vi "Configure Hardware.vi"(8 "error in (no error)":errorcluster, 11 "Hardware Resources in":T1={"AI"={"DAQmx Channel"="", "Max Input"=0.0, "Min Input"=0.0, "Sample Rate"=0.0, "DAQmx Task"="", "shunt resistor location"=-1, "external shunt resistor value"=249.0}, "AO"={"DAQmx Channel"="", "Max Output"=0.0, "Min Output"=0.0, "Sample Rate"=0.0, "DAQmx Task"=""}, "DO"={"DAQmx Channel"="", "Sample Rate"=0.0, "DAQmx Task"=""}, "DI"={"DAQmx Channel"="", "Sample Rate"=0.0, "DAQmx Task"=""}, "TC"={"DAQmx Channel"="", "Max Inout"=0.0, "Min Input"=0.0, "Sample Rate"=0.0, "DAQmx Task"="", "resistance configuration"=4, "r0"=100.0, "current excitation value"=0.0025, "current excitation source"=10167, "rtd type"=12481}} {"TC"."rtd type" items=["Pt3750"=12481, "Pt3851"=10071, "Pt3911"=12482, "Pt3916"=10069, "Pt3920"=10053, "Pt3928"=12483, "Custom"=10137]; "TC"."current excitation source" items=["Internal"=10200, "External"=10167, "None"=10230]; "TC"."resistance configuration" items=["2-Wire"=2, "3-Wire"=3, "4-Wire"=4]; "AI"."shunt resistor location" items=["default"=-1, "RSE"=10083, "NRSE"=10078, "Differential"=10106, "Pseudodifferential"=12529]}) -> (0 "error out":errorcluster, 3 "Hardware Resources out":T1={"AI"={"DAQmx Channel"="", "Max Input"=0.0, "Min Input"=0.0, "Sample Rate"=0.0, "DAQmx Task"="", "shunt resistor location"=-1, "external shunt resistor value"=249.0}, "AO"={"DAQmx Channel"="", "Max Output"=0.0, "Min Output"=0.0, "Sample Rate"=0.0, "DAQmx Task"=""}, "DO"={"DAQmx Channel"="", "Sample Rate"=0.0, "DAQmx Task"=""}, "DI"={"DAQmx Channel"="", "Sample Rate"=0.0, "DAQmx Task"=""}, "TC"={"DAQmx Channel"="", "Max Inout"=0.0, "Min Input"=0.0, "Sample Rate"=0.0, "DAQmx Task"="", "resistance configuration"=4, "r0"=100.0, "current excitation value"=0.0025, "current excitation source"=10167, "rtd type"=12481}} {"TC"."rtd type" items=["Pt3750"=12481, "Pt3851"=10071, "Pt3911"=12482, "Pt3916"=10069, "Pt3920"=10053, "Pt3928"=12483, "Custom"=10137]; "TC"."current excitation source" items=["Internal"=10200, "External"=10167, "None"=10230]; "TC"."resistance configuration" items=["2-Wire"=2, "3-Wire"=3, "4-Wire"=4]; "AI"."shunt resistor location" items=["default"=-1, "RSE"=10083, "NRSE"=10078, "Differential"=10106, "Pseudodifferential"=12529]})   [LabVIEW 2024, in "Acquisition.lvlib"]
doc: "Configure the hardware."
uses:
  Acquisition.lvlib
  Hardware Configuration.ctl
  <vilib>/DAQmx/configure/timing.llb/DAQmx Timing (Sample Clock).vi
  <vilib>/DAQmx/create/channels.llb/DAQmx Create Channel (DI-Digital Input).vi
  <vilib>/DAQmx/create/channels.llb/DAQmx Create Channel (AO-Current-Basic).vi
  <vilib>/DAQmx/create/channels.llb/DAQmx Create Channel (DO-Digital Output).vi
  <vilib>/DAQmx/create/channels.llb/DAQmx Create Channel (AI-Temperature-RTD).vi
  <vilib>/DAQmx/create/channels.llb/DAQmx Create Channel (AI-Current-Basic).vi
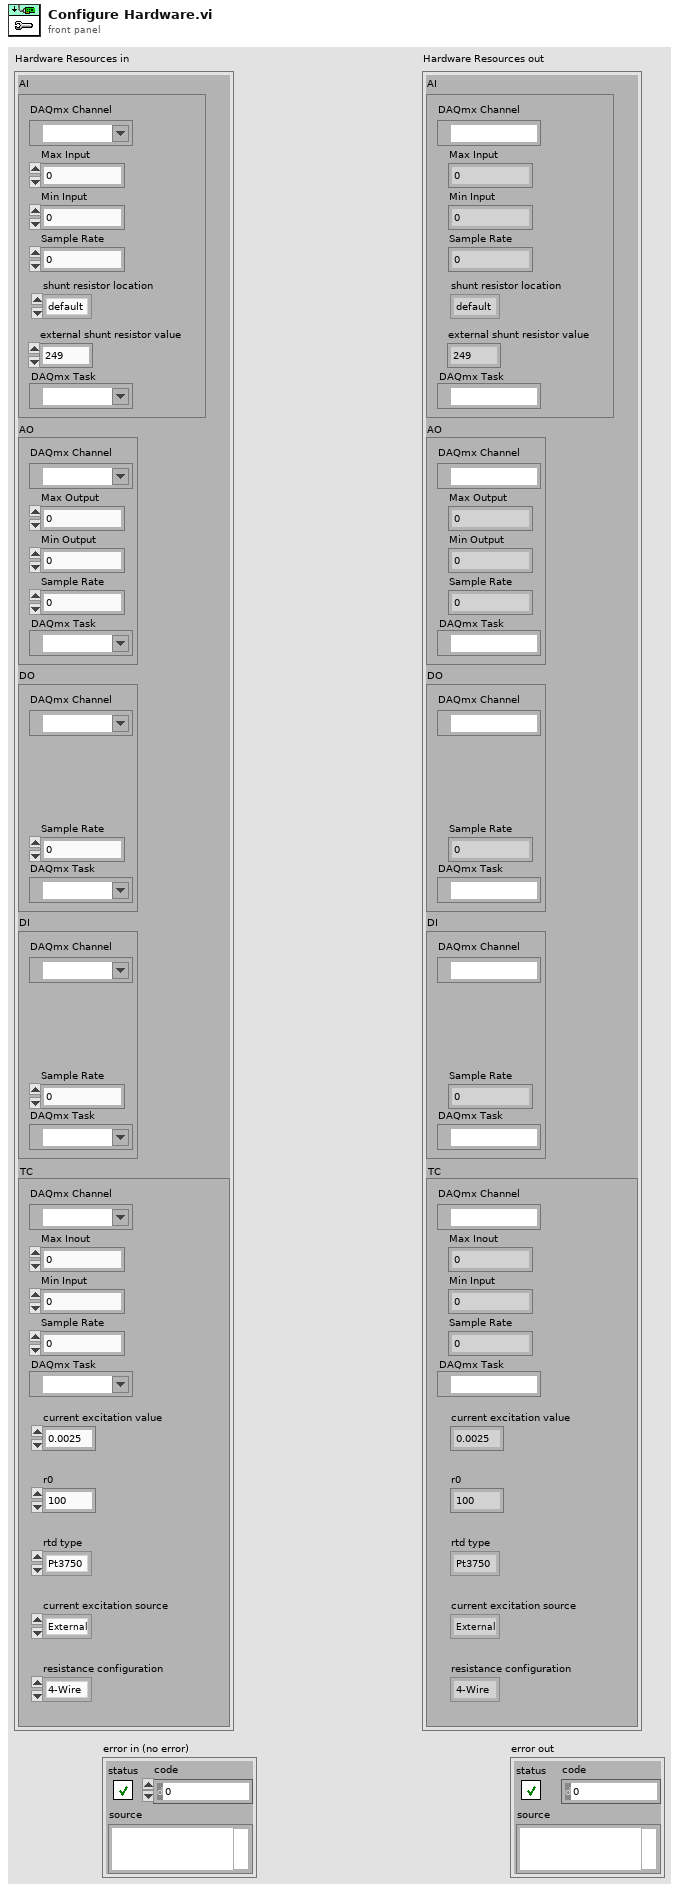
[diagram p1: front panel]
types:
  T1 = typedef "Acquisition.lvlib/Hardware Configuration.ctl" = cluster{"AI":cluster{"DAQmx Channel":tag, "Max Input":dbl, "Min Input":dbl, "Sample Rate":dbl, "DAQmx Task":refnum<k21>, "shunt resistor location":i32, "external shunt resistor value":dbl}, "AO":cluster{"DAQmx Channel":tag, "Max Output":dbl, "Min Output":dbl, "Sample Rate":dbl, "DAQmx Task":refnum<k21>}, "DO":cluster{"DAQmx Channel":tag, "Sample Rate":dbl, "DAQmx Task":refnum<k21>}, "DI":cluster{"DAQmx Channel":tag, "Sample Rate":dbl, "DAQmx Task":refnum<k21>}, "TC":cluster{"DAQmx Channel":tag, "Max Inout":dbl, "Min Input":dbl, "Sample Rate":dbl, "DAQmx Task":refnum<k21>, "resistance configuration":i32, "r0":dbl, "current excitation value":dbl, "current excitation source":i32, "rtd type":i32}}
  T2 = cluster{"DAQmx Channel":tag, "Max Input":dbl, "Min Input":dbl, "Sample Rate":dbl, "DAQmx Task":refnum<k21>, "shunt resistor location":i32, "external shunt resistor value":dbl}
  T3 = cluster{"DAQmx Channel":tag, "Max Output":dbl, "Min Output":dbl, "Sample Rate":dbl, "DAQmx Task":refnum<k21>}
  T4 = cluster{"DAQmx Channel":tag, "Sample Rate":dbl, "DAQmx Task":refnum<k21>}
  T5 = cluster{"DAQmx Channel":tag, "Max Inout":dbl, "Min Input":dbl, "Sample Rate":dbl, "DAQmx Task":refnum<k21>, "resistance configuration":i32, "r0":dbl, "current excitation value":dbl, "current excitation source":i32, "rtd type":i32}
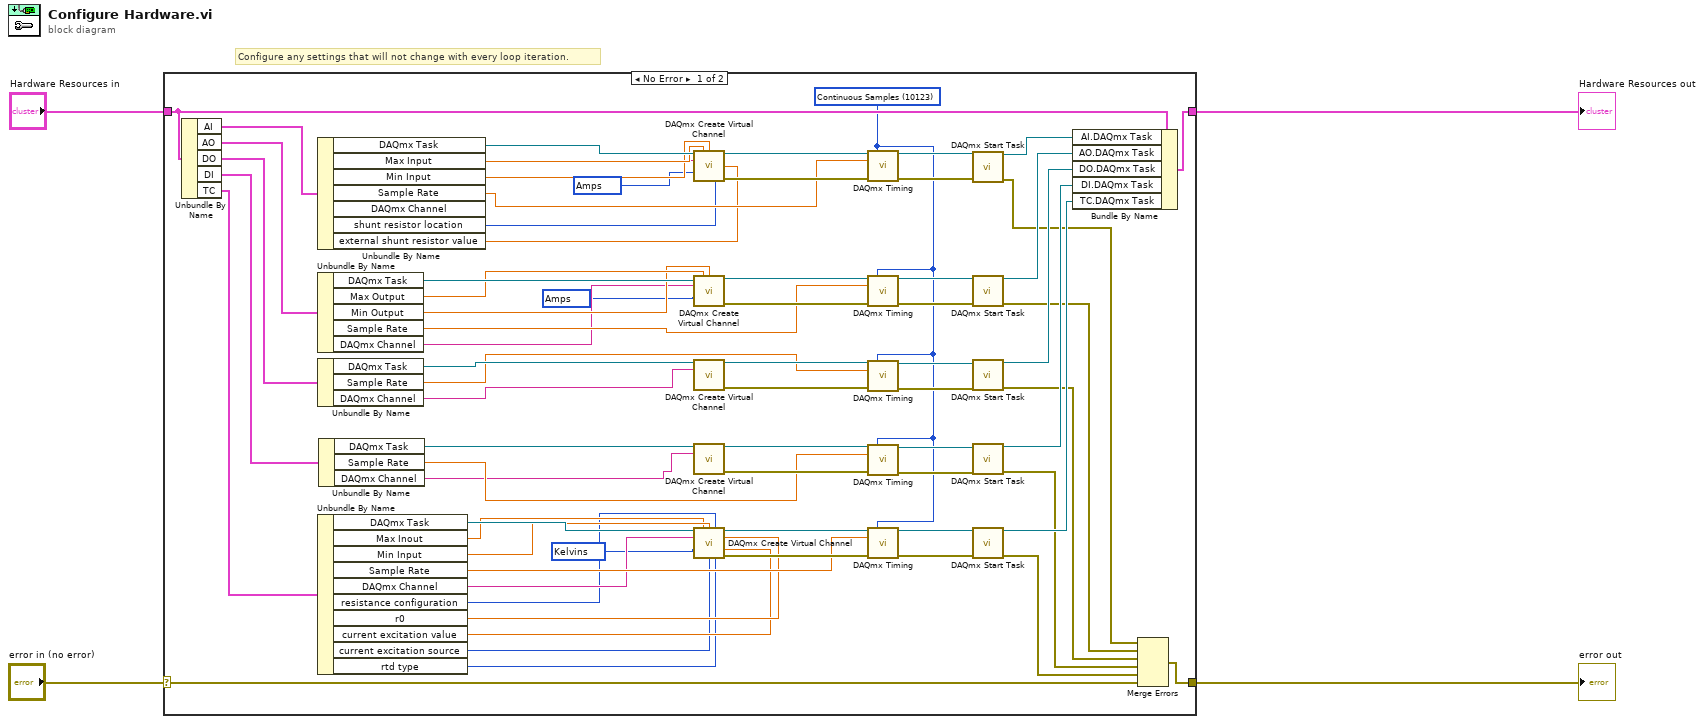
[diagram p0: block diagram]
diagram:
  # "Configure any settings that will not change with every loop iteration."
  n1 = case shown="No Error" "error in (no error)" {
    selector: "error in (no error)" -> [w59 w76]
    tunnel: [w8 w76] -> w3
    tunnel: "Hardware Resources in" -> [w53 w77]
    tunnel: [w75 w77] -> w2
    frame No Error {
      w5 = 10342 items=["Amps"=10342, "From Custom Scale"=10065] ("units")
      w6 = 10342 items=["Amps"=10342, "From Custom Scale"=10065] ("units")
      w7 = 10325 items=["Deg C"=10143, "Deg F"=10144, "Kelvins"=10325, "Deg R"=10145, "From Custom Scale"=10065] ("units")
      w14 = 10123 items=["Finite Samples"=10178, "Continuous Samples"=10123, "Hardware Timed Single Point"=12522] ("sample mode")
      n2 = Unbundle By Name(w53) -> ("AI"=w48:T2, "AO"=w49:T3, "DO"=w50:T4, "DI"=w51:T4, "TC"=w52:T5)
      n3 = Unbundle By Name(w48) -> ("DAQmx Task"=w37:refnum<k21>, "Max Input"=w32:dbl, "Min Input"=w31:dbl, "Sample Rate"=w30:dbl, "DAQmx Channel"=w29:tag, "shunt resistor location"=w28:i32, "external shunt resistor value"=w27:dbl)
      n4 = Unbundle By Name(w49) -> ("DAQmx Task"=w36:refnum<k21>, "Max Output"=w26:dbl, "Min Output"=w25:dbl, "Sample Rate"=w24:dbl, "DAQmx Channel"=w23:tag)
      n5 = Unbundle By Name(w50) -> ("DAQmx Task"=w35:refnum<k21>, "Sample Rate"=w22:dbl, "DAQmx Channel"=w21:tag)
      n6 = Unbundle By Name(w52) -> ("DAQmx Task"=w33:refnum<k21>, "Max Inout"=w17:dbl, "Min Input"=w18:dbl, "Sample Rate"=w16:dbl, "DAQmx Channel"=w15:tag, "resistance configuration"=w13:i32, "r0"=w12:dbl, "current excitation value"=w11:dbl, "current excitation source"=w10:i32, "rtd type"=w9:i32)
      n7 = Unbundle By Name(w51) -> ("DAQmx Task"=w34:refnum<k21>, "Sample Rate"=w20:dbl, "DAQmx Channel"=w19:tag)
      n8 = call-poly <vilib>:"DAQmx Create Virtual Channel.vi"("task in"=w37, "maximum value"=w32, "minimum value"=w31, "physical channels"=w29, "external shunt resistor value"=w27, "units"=w5, "shunt resistor location"=w28) -> ("task out"=w47:refnum<k21>, "error out"=w42:errorcluster)  [unwired: 7 in]
      n9 = call-poly <vilib>:"DAQmx Create Virtual Channel.vi"("task in"=w36, "maximum value"=w26, "minimum value"=w25, "physical channels"=w23, "units"=w6) -> ("task out"=w45:refnum<k21>, "error out"=w41:errorcluster)  [unwired: 9 in]
      n10 = call-poly <vilib>:"DAQmx Create Virtual Channel.vi"("task in"=w35, "lines"=w21) -> ("task out"=w44:refnum<k21>, "error out"=w40:errorcluster)  [unwired: 12 in]
      n11 = call-poly <vilib>:"DAQmx Create Virtual Channel.vi"("task in"=w34, "lines"=w19) -> ("task out"=w43:refnum<k21>, "error out"=w39:errorcluster)  [unwired: 12 in]
      n12 = call-poly <vilib>:"DAQmx Create Virtual Channel.vi"("task in"=w33, "maximum value"=w17, "minimum value"=w18, "resistance configuration"=w13, "physical channels"=w15, "r0"=w12, "units"=w7, "current excitation value"=w11, "current excitation source"=w10, "rtd type"=w9) -> ("task out"=w46:refnum<k21>, "error out"=w38:errorcluster)  [unwired: 4 in]
      n13 = call-poly <vilib>:"DAQmx Timing.vi"("task/channels in"=w47, "sample mode"=w14, "rate"=w30, "error in"=w42) -> ("task out"=w69:refnum<k21>, "error out"=w64:errorcluster)  [unwired: 10 in]
      n14 = call-poly <vilib>:"DAQmx Timing.vi"("task/channels in"=w45, "sample mode"=w14, "rate"=w24, "error in"=w41) -> ("task out"=w65:refnum<k21>, "error out"=w63:errorcluster)  [unwired: 10 in]
      n15 = call-poly <vilib>:"DAQmx Timing.vi"("task/channels in"=w44, "sample mode"=w14, "rate"=w22, "error in"=w40) -> ("task out"=w66:refnum<k21>, "error out"=w62:errorcluster)  [unwired: 10 in]
      n16 = call-poly <vilib>:"DAQmx Timing.vi"("task/channels in"=w43, "sample mode"=w14, "rate"=w20, "error in"=w39) -> ("task out"=w67:refnum<k21>, "error out"=w61:errorcluster)  [unwired: 10 in]
      n17 = call-poly <vilib>:"DAQmx Timing.vi"("task/channels in"=w46, "sample mode"=w14, "rate"=w16, "error in"=w38) -> ("task out"=w68:refnum<k21>, "error out"=w60:errorcluster)  [unwired: 10 in]
      n18 = call <vilib>:"DAQmx Start Task.vi"("task/channels in"=w69, "error in"=w64) -> ("task out"=w74:refnum<k21>, "error out"=w54:errorcluster)  [unwired: 12 in]
      n19 = call <vilib>:"DAQmx Start Task.vi"("task/channels in"=w65, "error in"=w63) -> ("task out"=w73:refnum<k21>, "error out"=w55:errorcluster)  [unwired: 12 in]
      n20 = call <vilib>:"DAQmx Start Task.vi"("task/channels in"=w66, "error in"=w62) -> ("task out"=w72:refnum<k21>, "error out"=w56:errorcluster)  [unwired: 12 in]
      n21 = call <vilib>:"DAQmx Start Task.vi"("task/channels in"=w67, "error in"=w61) -> ("task out"=w71:refnum<k21>, "error out"=w57:errorcluster)  [unwired: 12 in]
      n22 = call <vilib>:"DAQmx Start Task.vi"("task/channels in"=w68, "error in"=w60) -> ("task out"=w70:refnum<k21>, "error out"=w58:errorcluster)  [unwired: 12 in]
      n23 = Bundle By Name(cluster=w53, "AI.DAQmx Task"=w74, "AO.DAQmx Task"=w73, "DO.DAQmx Task"=w72, "DI.DAQmx Task"=w71, "TC.DAQmx Task"=w70) -> (w75:T1)
      n24 = Merge Errors(w54, w55, w56, w57, w58, w59) -> (w8:errorcluster)
    }
    frame Error {
    }
  }
  "Hardware Resources out" <- w2
  "error out" <- w3
